vi "Open_file.vi"(6 "error in":errorcluster, 8 "File Name input":string="stamtest.pdf ", 9 "Work-Place path\n(with the webarch.exe)":path) -> (0 "error out":errorcluster)   [LabVIEW 2017]
panel:
  out "File Name":string="webarch "
  in  "wait until completion? (T)":bool
  in  "run minimized? (F)":bool=TRUE
  out "standard output":string
  out "standard error":string
  out "return code":i32
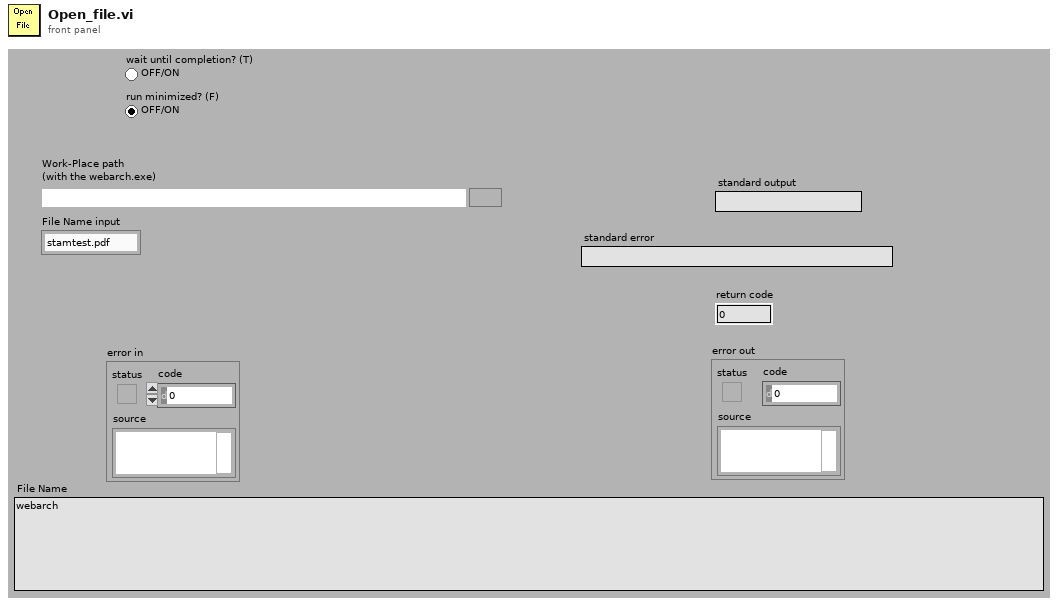
[diagram p1: front panel]
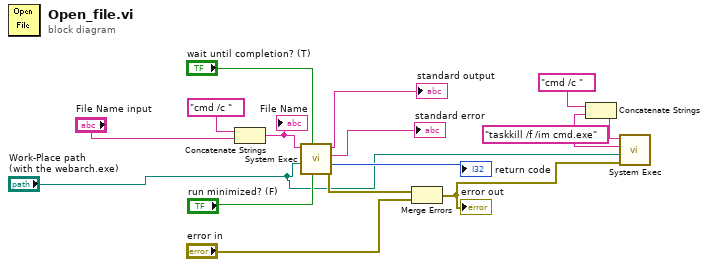
[diagram p0: block diagram]
diagram:
  w1 = "taskkill /f /im cmd.exe" ("string")
  n1 = Concatenate Strings("cmd /c " ("File Name"), "File Name input") -> (w6:string)
  "File Name" <- w6
  n2 = call <vilib>:"System Exec.vi"("run minimized? (F)"="run minimized? (F)", "wait until completion? (T)"="wait until completion? (T)", "working directory"="Work-Place path\n(with the webarch.exe)", "command line"=w6) -> ("error out"=w10:errorcluster, "return code"=→"return code":i32, "standard error"=→"standard error":string, "standard output"=→"standard output":string)  [unwired: 4 in]
  n3 = Merge Errors(w10, "error in") -> (w3:errorcluster)
  "error out" <- w3
  n4 = Concatenate Strings("cmd /c " ("File Name"), w1) -> (w4:string)
  n5 = call <vilib>:"System Exec.vi"("error in (no error)"=w3, "working directory"="Work-Place path\n(with the webarch.exe)", "standard input"=w1, "command line"=w4) -> ()  [unwired: 4 in, 4 out]
